vi "Generate_Sound_Example.vi"() -> ()   [LabVIEW 2011]
doc: "This VI illustrates how to generate and play sine, square, sawtooth and triangle waveforms. You can change the frequency and type of the waveform generated as it plays continuously."
uses:
  <vilib>/sound2/lvsound2.llb/Sound Data Format.ctl
  <vilib>/sound2/lvsound2.llb/Sampling Mode.ctl
  <vilib>/sound2/lvsound2.llb/Sound Output Set Volume (Single).vi
  <vilib>/sound2/lvsound2.llb/Sound Output Write (DBL Single).vi
  <vilib>/measure/NI_MABase.lvlib
panel:
  out "Numeric":i32
  in  "Sound Format":T1={"sample rate (S/s)"=44100.0, "number of channels"=2, "bits per sample"=16}
  in  "Volume":dbl(slide)=70.40816326530613 scale=0.0..100.0
  out "Generated Sound":waveform(dbl)(graph)={"t0"=timestamp(1.2471655328798186 s since 1904-01-01), "dt"=2.2675736961451248e-05, "Y"=[]}
  in  "Waveform Type":enum16{"Sine", "Square", "Sawtooth", "Triangle"}(ring)
  in  "Frequency":dbl=500.0 format="%0.2p"
  in  "stop":bool
  in  "Number of Samples/ch":i32=5000
  in  "Device ID":u32
  # "This VI illustrates how to generate and play sine, square, sawtooth and triangle waveforms continuously. \n\nInstructions to execute the VI:\n1.  Specify Device ID, bits per sample, sample rate and number of samples (buffer size).\n2.  Select the waveform type to play and its initial frequency.\n3.  Run the VI. Waveforms are generated and sent to both the graph and your speakers.\n3.  Change the frequency to change the pitch of the sound.\n4.  Change the waveform type to start playing differently shaped waves.\n5.  Press the stop button when done."
  # "Configuration"
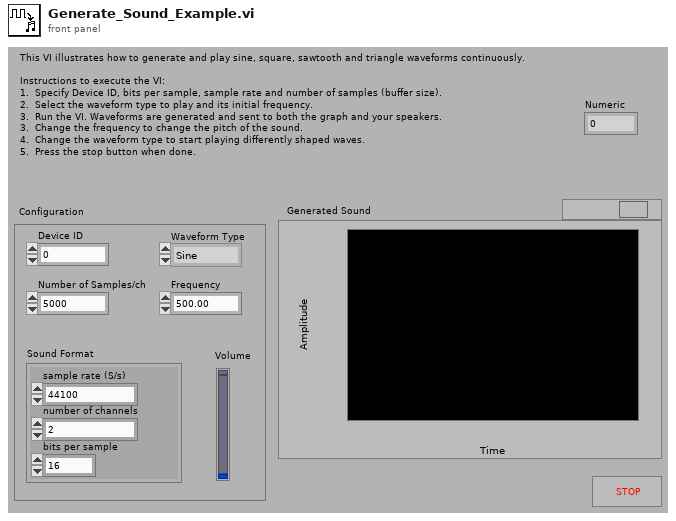
[diagram p1: front panel]
types:
  T1 = typedef "Sound Data Format.ctl" = cluster{"sample rate (S/s)":dbl, "number of channels":i32, "bits per sample":i32}
  T2 = typedef "Sampling Mode.ctl" = i32
  T3 = typedef "Sound Output Task ID.ctl" = u32
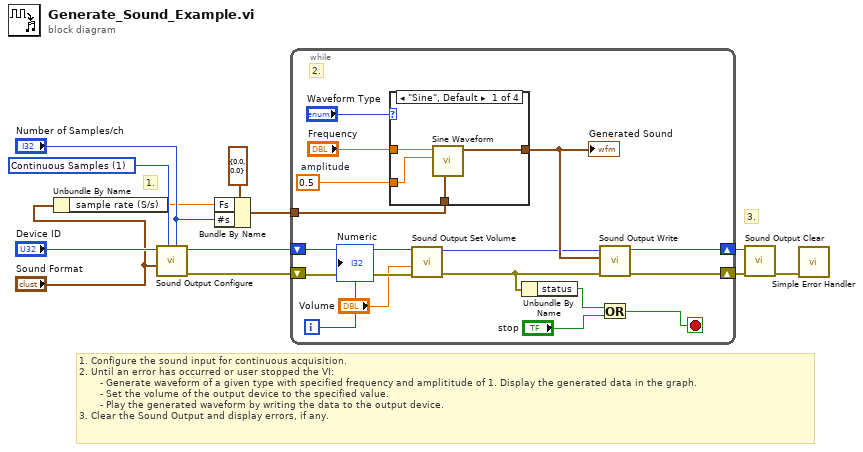
[diagram p0: block diagram]
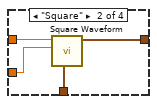
[diagram p2: hidden frame]
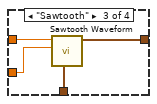
[diagram p3: hidden frame]
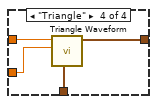
[diagram p4: hidden frame]
diagram:
  w7 = T2 1 items=["Finite Samples", "Continuous Samples"] ("sample mode")
  # "3."
  # "1."
  # "1. Configure the sound input for continuous acquisition.\n2. Until an error has occurred or user stopped the VI: \n      \t- Generate waveform of a given type with specified frequency and amplititude of 1. Display the generated data in the graph. \n       - Set the volume of the output device to the specified value.\n      \t- Play the generated waveform by writing the data to the output device.\n3. Clear the Sound Output and display errors, if any."
  n1 = Unbundle By Name("Sound Format") -> ("sample rate (S/s)"=w2:dbl)
  n2 = call <vilib>:"Sound Output Configure.vi"("number of samples/ch"="Number of Samples/ch", "sample mode"=w7, "sound format"="Sound Format", "device ID"="Device ID") -> ("error out"=w12:errorcluster, "task ID"=w11:T3)  [unwired: 6 in]
  n3 = Bundle By Name(cluster=cluster{"Fs":dbl, "#s":dbl} {"Fs"=0.0, "#s"=0.0} ("sampling info"), "Fs"=w2, "#s"="Number of Samples/ch") -> (w4:cluster{"Fs":dbl, "#s":dbl})
  n4 = while {
    shift-right: [w27] -> w10
    shift-left: w12 -> [w18]
    shift-right: [w28] -> w9
    shift-left: w11 -> [w16]
    tunnel: w4 -> [w23]
    i -> [w14]
    stop <- w13 stop-if-true
    w21 = 0.5  # amplitude
    # "2."
    n5 = case shown="\"Sine\", Default" "Waveform Type" {
      tunnel: "Frequency" -> [w32 w35 w37 w44]
      tunnel: [w31 w34 w39 w43] -> w20
      tunnel: w23 -> [w30 w36 w40 w42]
      tunnel: w21 -> [w29 w33 w38 w41]
      frame "Sine", Default {
        n6 = call <vilib>:"Sine Waveform.vi"("sampling info"=w30, "amplitude"=w29, "frequency"=w32) -> ("signal out"=w31:waveform(dbl))  [unwired: 7 in, 1 out]
      }
      frame "Square" {
        n7 = call <vilib>:"Square Waveform.vi"("sampling info"=w36, "amplitude"=w33, "frequency"=w35) -> ("signal out"=w34:waveform(dbl))  [unwired: 7 in, 1 out]
      }
      frame "Sawtooth" {
        n8 = call <vilib>:"Sawtooth Waveform.vi"("sampling info"=w40, "amplitude"=w38, "frequency"=w37) -> ("signal out"=w39:waveform(dbl))  [unwired: 7 in, 1 out]
      }
      frame "Triangle" {
        n9 = call <vilib>:"Triangle Waveform.vi"("sampling info"=w42, "amplitude"=w41, "frequency"=w44) -> ("signal out"=w43:waveform(dbl))  [unwired: 7 in, 1 out]
      }
    }
    "Generated Sound" <- w20
    n10 = call-poly <vilib>:"Sound Output Set Volume.vi"("error in (no error)"=w18, "volume"="Volume", "task ID"=w16) -> ("error out"=w19:errorcluster, "task ID out"=w17:T3)  [unwired: 7 in]
    n11 = Unbundle By Name(w19) -> ("status"=w24:bool)
    n12 = call-poly <vilib>:"Sound Output Write.vi"("error in (no error)"=w19, "data"=w20, "task ID"=w17) -> ("error out"=w27:errorcluster, "task ID out"=w28:T3)  [unwired: 7 in]
    n13 = Or(x=w24, y="stop") -> (x .or. y?=w13:bool)
    "Numeric" <- w14
  }
  n14 = call <vilib>:"Sound Output Clear.vi"("error in (no error)"=w10, "task ID"=w9) -> ("error out"=w3:errorcluster)  [unwired: 9 in]
  n15 = call <vilib>:"Simple Error Handler.vi"("error in (no error)"=w3) -> ()  [unwired: 4 in, 5 out]
